vi "Initialize-UI-elements.vi"(8 "error in (no error)":errorcluster, 10 "Main VI ref":refnum<vi>, 11 "Object ref in":T1) -> (0 "error out":errorcluster, 3 "Object ref out":T1)   [LabVIEW 2013, in "PowderDeposition.lvlib" / "PD-Main.lvclass"]
uses:
  PD-Main.lvclass
  Object-reference.ctl
  UI-references.ctl
  UI-elements.ctl
  PD-Main.lvclass/PD-Main.ctl
panel:
  out "Elements":string[](array[string])
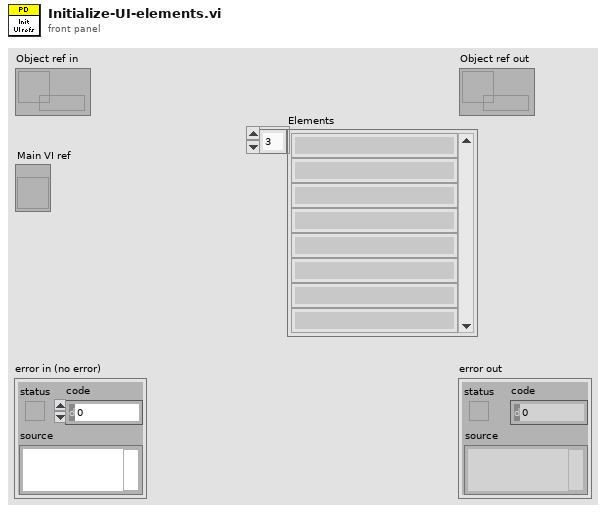
[diagram p1: front panel]
types:
  T1 = typedef "PowderDeposition.lvlib/PD-Main.lvclass/Object-reference.ctl" = refnum<data-value>
  T2 = typedef "PowderDeposition.lvlib/PD-Main.lvclass/UI-references.ctl" = cluster{"Motors-selection":refnum<vi>, "Motors-status":refnum<vi>, "Available-actions":refnum<vi>, "Options":refnum<vi>, "Motor sequences":refnum<vi>[], "Client status":refnum<vi>}
  T3 = typedef "PowderDeposition.lvlib/PD-Main.lvclass/UI-elements.ctl" = enum16{"Motors-selection", "Motors-status", "Status", "Options", "Available-actions", "M1-sequence", "M2-sequence", "M3-sequence", "M4-sequence"}
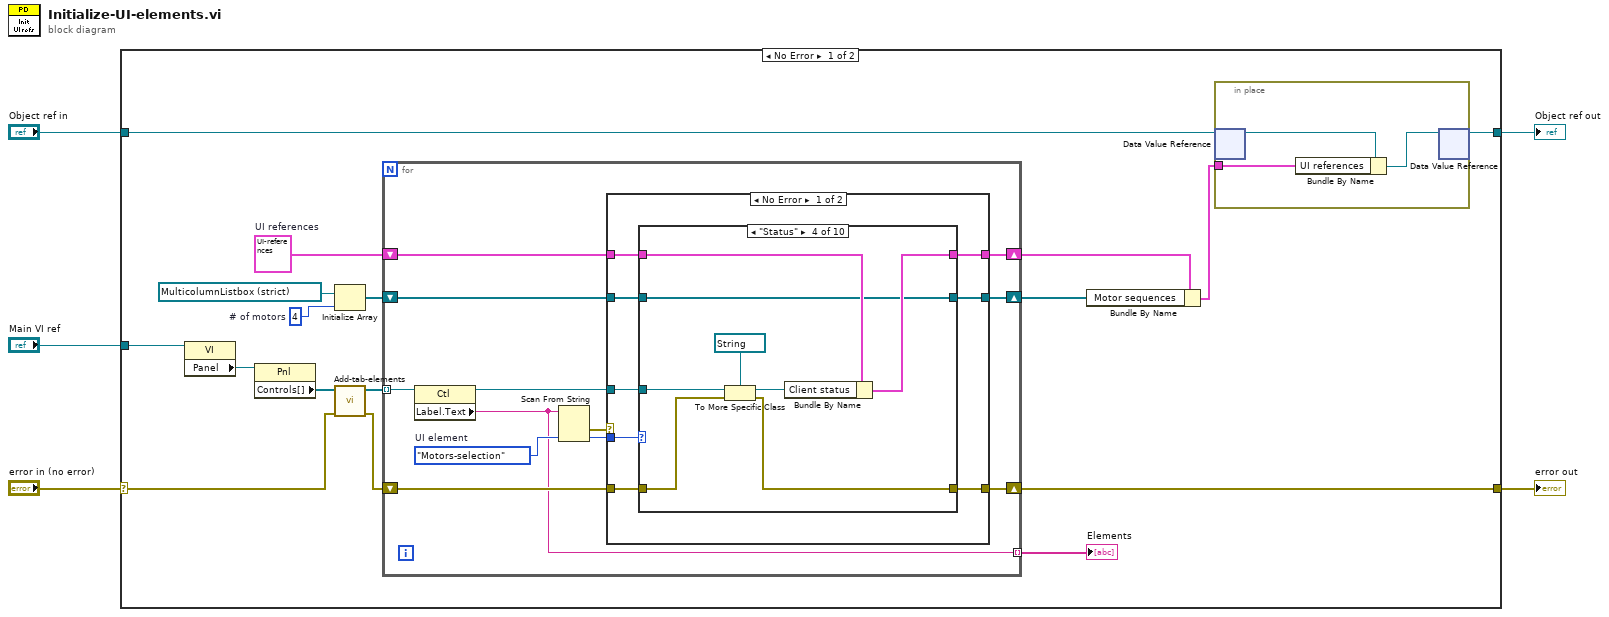
[diagram p0: block diagram]
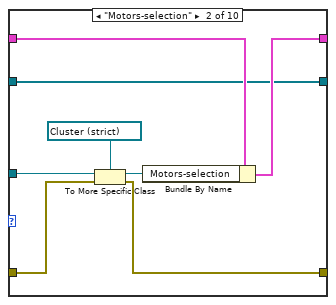
[diagram p3: hidden frame]
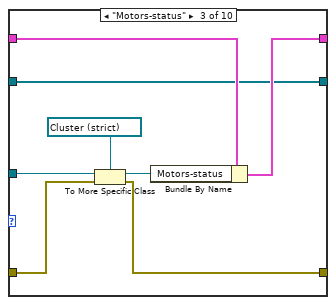
[diagram p4: hidden frame]
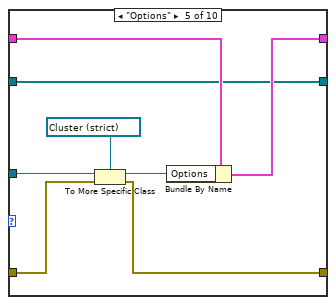
[diagram p5: hidden frame]
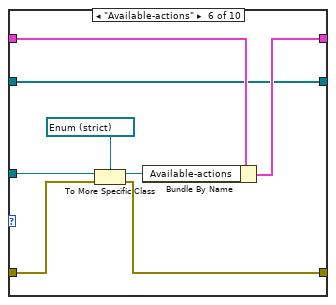
[diagram p6: hidden frame]
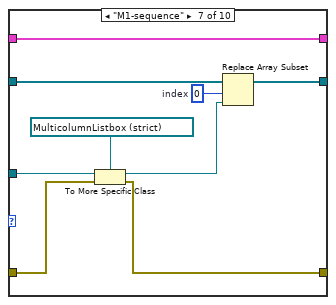
[diagram p7: hidden frame]
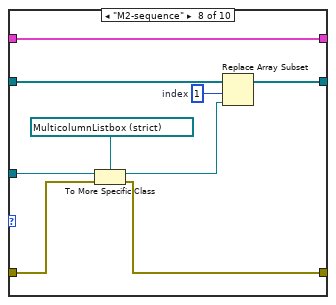
[diagram p8: hidden frame]
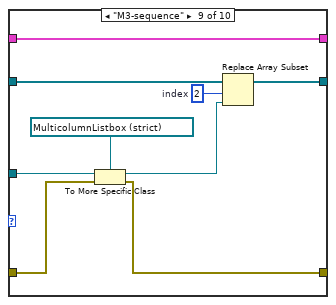
[diagram p9: hidden frame]
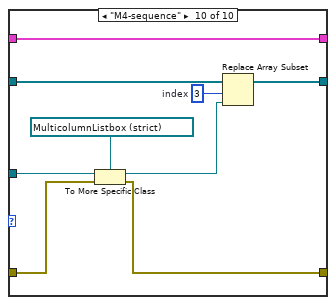
[diagram p10: hidden frame]
diagram:
  n1 = case shown="No Error" "error in (no error)" {
    selector: "error in (no error)" -> [w7 w129]
    tunnel: [w16 w129] -> w4
    tunnel: [w21 w128] -> w2
    tunnel: "Object ref in" -> [w22 w128]
    tunnel: "Main VI ref" -> [w20 _]
    frame No Error {
      w14 = 4  # # of motors
      w18 = T2 {"Motors-selection"=refnum, "Motors-status"=refnum, "Available-actions"=refnum, "Options"=refnum, "Motor sequences"=[], "Client status"=refnum}  # UI references
      n2 = property class="VI"(reference=w20) -> ("Panel"=w19:refnum<vi>)  [unwired: 1 in, 2 out]
      n3 = property class="Pnl"(reference=w19) -> ("Controls[]"=w9:refnum<vi>[])  [unwired: 1 in, 2 out]
      n4 = Initialize Array(refnum<vi> refnum ("M1-sequence"), w14) -> (w13:refnum<vi>[])
      n5 = call "Add-tab-elements.vi"("error in (no error)"=w7, "Controls in"=w9) -> ("error out"=w6:errorcluster, "Controls out"=w8:refnum<vi>[])  [unwired: 8 in]
      n6 = for {
        tunnel: w8 -> [w34] mode=indexing
        shift-right: [w28] -> w17
        shift-left: w18 -> [w31]
        shift-right: [w26] -> w16
        shift-left: w6 -> [w27]
        shift-right: [w24] -> w11
        shift-left: w13 -> [w25]
        tunnel: [w23] -> w10 mode=indexing
        w33 = UI-elements."Motors-selection"  # UI element
        n7 = property class="Ctl"(reference=w34) -> (reference out=w29:refnum<vi>, "Label.Text"=w23:string)  [unwired: 1 in, 1 out]
        n8 = Scan From String(input string=w23, default 1=w33) -> (error out=w32:errorcluster, output 1=w30:T3)  [unwired: 3 in, 2 out]
        n9 = case shown="No Error" w32 {
          tunnel: w31 -> [w42 w124]
          tunnel: w30 -> [w41 _]
          tunnel: w29 -> [w40 _]
          tunnel: [w39 w124] -> w28
          tunnel: w27 -> [w38 w122]
          tunnel: [w37 w122] -> w26
          tunnel: w25 -> [w36 w123]
          tunnel: [w35 w123] -> w24
          frame No Error {
            n10 = case shown="\"Status\"" w41 {
              tunnel: w42 -> [w45 w53 w61 w69 w77 w85 w90 w99 w108 w117]
              tunnel: w40 -> [_ w51 w59 w67 w75 w83 w94 w103 w112 w121]
              tunnel: [w45 w52 w60 w68 w76 w84 w90 w99 w108 w117] -> w39
              tunnel: w38 -> [w44 w50 w58 w66 w74 w82 w93 w102 w111 w120]
              tunnel: [w44 w49 w57 w65 w73 w81 w92 w101 w110 w119] -> w37
              tunnel: w36 -> [w43 w46 w54 w62 w70 w78 w89 w98 w107 w116]
              tunnel: [w43 w46 w54 w62 w70 w78 w88 w97 w106 w115] -> w35
              frame Default {
              }
              frame "Motors-selection" {
                n11 = To More Specific Class(target class=refnum<vi> refnum ("Motors-selection"), reference=w51, error in=w50) -> (specific class reference=w47:refnum<vi>, error out=w49:errorcluster)
                n12 = Bundle By Name(cluster=w53, "Motors-selection"=w47) -> (w52:T2)
              }
              frame "Motors-status" {
                n13 = To More Specific Class(target class=refnum<vi> refnum ("Motors-status"), reference=w59, error in=w58) -> (specific class reference=w55:refnum<vi>, error out=w57:errorcluster)
                n14 = Bundle By Name(cluster=w61, "Motors-status"=w55) -> (w60:T2)
              }
              frame "Status" {
                n15 = To More Specific Class(target class=refnum<vi> refnum ("Motors-status"), reference=w67, error in=w66) -> (specific class reference=w63:refnum<vi>, error out=w65:errorcluster)
                n16 = Bundle By Name(cluster=w69, "Client status"=w63) -> (w68:T2)
              }
              frame "Options" {
                n17 = To More Specific Class(target class=refnum<vi> refnum ("Options"), reference=w75, error in=w74) -> (specific class reference=w71:refnum<vi>, error out=w73:errorcluster)
                n18 = Bundle By Name(cluster=w77, "Options"=w71) -> (w76:T2)
              }
              frame "Available-actions" {
                n19 = To More Specific Class(target class=refnum<vi> refnum ("Available-actions"), reference=w83, error in=w82) -> (specific class reference=w79:refnum<vi>, error out=w81:errorcluster)
                n20 = Bundle By Name(cluster=w85, "Available-actions"=w79) -> (w84:T2)
              }
              frame "M1-sequence" {
                w87 = 0  # index
                n21 = To More Specific Class(target class=refnum<vi> refnum ("M1-sequence"), reference=w94, error in=w93) -> (specific class reference=w86:refnum<vi>, error out=w92:errorcluster)
                n22 = Replace Array Subset(array=w89, new element=w86, index=w87) -> (w88:refnum<vi>[])
              }
              frame "M2-sequence" {
                w96 = 1  # index
                n23 = To More Specific Class(target class=refnum<vi> refnum ("M1-sequence"), reference=w103, error in=w102) -> (specific class reference=w95:refnum<vi>, error out=w101:errorcluster)
                n24 = Replace Array Subset(array=w98, new element=w95, index=w96) -> (w97:refnum<vi>[])
              }
              frame "M3-sequence" {
                w105 = 2  # index
                n25 = To More Specific Class(target class=refnum<vi> refnum ("M1-sequence"), reference=w112, error in=w111) -> (specific class reference=w104:refnum<vi>, error out=w110:errorcluster)
                n26 = Replace Array Subset(array=w107, new element=w104, index=w105) -> (w106:refnum<vi>[])
              }
              frame "M4-sequence" {
                w114 = 3  # index
                n27 = To More Specific Class(target class=refnum<vi> refnum ("M1-sequence"), reference=w121, error in=w120) -> (specific class reference=w113:refnum<vi>, error out=w119:errorcluster)
                n28 = Replace Array Subset(array=w116, new element=w113, index=w114) -> (w115:refnum<vi>[])
              }
            }
          }
          frame Error {
          }
        }
      }
      "Elements" <- w10
      n29 = Bundle By Name(cluster=w17, "Motor sequences"=w11) -> (w12:T2)
      n30 = in-place {
        in-place-border: w12 -> [w125]
        n31 = in-place-dvr #1(w22) -> (w127:refnum<class "PD-Main.lvclass">)  [unwired: 1 out]
        n32 = Bundle By Name(cluster=w127, "UI references"=w125) -> (w126:refnum<class "PD-Main.lvclass">)
        n33 = in-place-dvr #1(w126) -> (w21:T1)  [unwired: 1 out]
      }
    }
    frame Error {
    }
  }
  "error out" <- w4
  "Object ref out" <- w2
